vi "Load IBW File.vi"(2 "Page":i32=1, 3 "file path (dialog if empty)":path=path "Q:/inst/AFM Drift/SAA00010002.ibw") -> (0 "Image":T1(plugin-control), 1 "Wave Note":string="ScanSize: 4e-06\rFastScanSize: 4e-06\rSlowScanSize: 4e-06\rScanRate: 1.0016\rXOffset: -4.35e-06\rYOffset: -8.3777e-06\rPointsLines: 128\rScanPoints: 128\rScanLines: 128\rScanAngle: 0\rImagingMode:Contact\rInvOLS: 1e-07\rSpringConstant: 1\rAmpInvOLS: 1.09e-07\rFastRatio: 1\rSlowRatio: 1\rTopLine: 255\rBottomLine: 0\rScanMode:Closed Loop\rNapMode:Off\rFMapScanTime: 17.231\rFMapScanPoints: 32\rFMapScanLines: 32\rFMapXYVelocity: 8e-05\rFMapBookWise: 0\rChannel1DataType: 1\rDataTypeSum: 21\rPhaseOffset: 123.8\rPhaseOffset1: 0\rNapPhaseOffset: 123.8\rVoltageParm: 0\rNapParms: 0\r32 bit channel:Height\rReal Parms: End\rInitial Parms: Start\rScanSize: 4e-06\rFastScanSize: 4e-06\rSlowScanSize: 4e-06\rScanRate: 1.0016\rScanSpeed: 1.0016e-05\rXOffset: -4.35e-06\rYOffset: -8.3777e-06\rScanPoints: 128\rScanLines: 128\rRoundFactor: 0.04\rIntegralGain: 48.62\rProportionalGain: 0\rScanAngle: 0\rScanAngleFactor: 1\rAmplitudeSetpointVolts: 0.54\rAmplitudeSetpointMeters: 1e-08\rDriveAmplitude: 6.4121\rDriveFrequency: 49841\rSweepWidth: 5000\rSlowScanEnabled: 1\rDeflectionSetpointVolts: -0.04\rDeflectionSetpointMeters: 0\rDeflectionSetpointNewtons: 5e-09\rImagingMode: 0\rMaxScanSize: 9e-05\rInvOLS: 1e-07\rSpringConstant: 1\rDisplaySpringConstant: 1e-09\rScanStateChanged: 0\rScanDown: 1\rXLVDTSens: 7.5725e-06\rYLVDTSens: 7.2348e-06\rZLVDTSens: 1.3012e-06\rXLVDTOffset: -0.34\rYLVDTOffset: -0.51\rZLVDTOffset: 0\rYIgain: 8.55\rYPgain: -inf\rXIgain: 8.9531\rXPgain: -inf\rLastScan: 0\rXPiezoSens: 3.8579e-07\rYPiezoSens: 3.9432e-07\rZPiezoSens: 6.8805e-08\rXDriveOffset: 0\rYDriveOffset: 0\rSweepPoints: 480\rSecretGain: 0\rYSgain: 10.5\rXSgain: 10.95\rDIsplayLVDTTraces: 0\rPhaseOffset: 123.8\rBaseSuffix: 2\rSaveImage: 2\rParmChange: 0\rADCgain: 0\rOldADCgain: 12\rOldScanSize: NaN\rOldYOffset: -8.3777e-06\rOldXOffset: -4.3966e-06\rZIgain: 10.15\rZPgain: -inf\rZSgain: 0\rAmpInvOLS: 1.09e-07\rUpdateCounter: 0\rDoMunge: 0\rXMungeAlpha: 1\rYMungeAlpha: 1\rZMungeAlpha: 1\rStartHeadTemp: 33.375 °C\rStartScannerTemp: 26.938 °C\rHas1xACDeflGain: 1\rDontChangeXPT: 0\rLowNoise: 1\rScreenRatio: 0.75\rXDriftRate: 0\rYDriftRate: 0\rXDriftTotal: 0\rYDriftTotal: 0\rDriftBIts: 0\rDriftCount: 0\rSetpoint: 0.0008\rFastRatio: 1\rSlowRatio: 1\rTopLine: 255\rBottomLine: 0\rScanStatus: 1\rIs1DPlus: 0\rDelayUpdate: 0\rMarkerRatio: 0\rStartLineCount: 128\rOldAmplitudeSetpointVolts: 0.54\rOldDeflectionSetPointVolts: 0\rScanMode: 0\rInterpolate: -624\rTipVoltage: 0\rStartHeaterTemp: 0 °C\rEndHeaterTemp: 0\rSurfaceVoltage: 0\rFreqIgain: 5\rFreqPgain: 0\rFreqSgain: 0\rOrcaGain: NaN\rFreqGainOn: 0\rUserIn0Gain: 1\rUserIn1Gain: 1\rUserIn2Gain: 1\rLateralGain: 1\rIsBipolar: 0\rFrequencyHack: 0\rMagneticField: 0\rDriveGainOn: 0\rDriveIGain: 0\rDrivePGain: 0\rDriveSGain: 0\rUserIn0Offset: 0\rUserIn1Offset: 0\rUserIn2Offset: 0\rLateralOffset: 0\rLastImage: 0\rZoomSize: 0\rZoomXOffset: -4.3966e-06\rZoomYOffset: -8.3777e-06\rUser0Voltage: 0\rUser1Voltage: 0\rExtendedZ: 0\rDriveAmplitude1: 0.1\rDriveFrequency1: 0\rSweepWidth1: 5000\rPhaseOffset1: 0\rAmp2InvOLS: 2e-08\rVoltageParm: 0\rMicroscopeID: 3\rCapacitanceSens: 1\rCapacitanceOffset: 0\rCapPhaseOffset: 0\rTipBiasOffset: 0\rTipHeaterOffset: 0\rSurfaceBiasOffset: 0\rUseCantHolder: 0\rCurrentCantHolder: 2\rHasClickRing: 0\rXScanDirection: 1\rYScanDirection: 1\rSaveImageCount: 0\rSaveImageLines: 64\rOrcaGain2: NaN\rUpdateSlowWave: 0\rFBFilterBW: 1000\rCurrentSetpointAmps: 1\rCurrentSetpointVolts: 1\rOldCurrentSetpointVolts: 1\rOldCurrentSetpointAmps: 1\rHasFM: 1\rLastScanWithdraw: 1\rHasLaserRelay: 0\rToggleLaserRelay: 0\rDecimation: 156\rDARTIGain: 5.5\rDARTPGain: 0\rSampleHolder: 1\rManualSampleHolder: 0\rCypherXPTLock: 0\rXPTLock: 2048\rLogFeedback: 0\rARSysScanBusy: 0\rSimpleControls: 0\rPointsLines: 128\rFreeAirAmplitude: NaN\rFreeAirPhase: NaN\rFreeAirDeflection: -0.14617\rFreeAirDriveAmplitude: 0\rContinualRetune: 0\rForceFilter: 0\rTemperatureSens: 1\rTemperatureOffset: 0\rOffsetBehavior: 0\rInputRange: 10\rXLVDTSensSlope: 0\rYLVDTSensSlope: 0\rXLVDTSensIntercept: 0\rYLVDTSensIntercept: 0\rHaveWeKilledTheProgressBar: 0\rPreScanSetting: 0\rImageFrameTime: 0\rMicroscopeModel:MFP3D\rInitial Parms: End\rNapIntegralGain: 10\rNapProportionalGain: 0\rNapDeflectionSetpointVolts: 0.5\rNapAmplitudeSetpointVolts: 0.8\rNapDissipationSetpointVolts: 0.2\rNapFrequencySetPointHz: 0\rNapCurrentSetpointAmps: 1\rNapDriveAmplitude: 1\rNapDriveFrequency: 49797\rNapDriveAmplitude1: 0.1\rNapDriveFrequency1: 4.2e+05\rNapPhaseOffset: 90\rNapTipVoltage: 3\rNapSurfaceVoltage: 0\rNapUser0Voltage: 0\rNapUser1Voltage: 0\rNapHeight: 5e-08\rNapStartHeight: 0\rNapTime: 0.10016\rNapMode: 0\rNapParms: 0\rPotentialIGain: 3\rPotentialPGain: 0\rPotentialGainOn: 0\rElectricTune: 0\rNapCurrentSetpointVolts: 1\rPotentialLoopLimit: 9\rChannel1DataType: 1\rChannel2DataType: 3\rChannel3DataType: 5\rChannel4DataType: 0\rChannel5DataType: 0\rChannel6DataType: 0\rDataTypeSum: 21\rChannel1Show: 2\rChannel2Show: 2\rChannel3Show: 2\rChannel4Show: 2\rChannel5Show: 2\rChannel6Show: 1\rChannelShowSum: 7\rRealPlanefit: 2\rSavePlanefit: 0\rHeightCapture: 2\rHeight1DataScale: 1.2e-09\rHeight1DataOffset: 0\rHeight1RealPlanefit: 2\rHeight1SavePlanefit: 4\rHeight1ColorMap: 2\rHeight2DataScale: 5e-08\rHeight2DataOffset: 0\rHeight2RealPlanefit: 2\rHeight2SavePlanefit: 2\rHeight2ColorMap: 1\rDeflectionCapture: 2\rDeflection1DataScale: 1e-08\rDeflection1DataOffset: 0\rDeflection1RealPlanefit: 1\rDeflection1SavePlanefit: 0\rDeflection1ColorMap: 1\rDeflection2DataScale: 1e-08\rDeflection2DataOffset: 0\rDeflection2RealPlanefit: 2\rDeflection2SavePlanefit: 2\rDeflection2ColorMap: 1\rAmplitudeCapture: 2\rAmplitude1DataScale: 1.5e-10\rAmplitude1DataOffset: -0\rAmplitude1RealPlanefit: 1\rAmplitude1SavePlanefit: 0\rAmplitude1ColorMap: 9\rAmplitude2DataScale: 2e-08\rAmplitude2DataOffset: 0\rAmplitude2RealPlanefit: 1\rAmplitude2SavePlanefit: 2\rAmplitude2ColorMap: 1\rZSensorCapture: 2\rZSensor1DataScale: 8.4e-08\rZSensor1DataOffset: -0\rZSensor1RealPlanefit: 4\rZSensor1SavePlanefit: 2\rZSensor1ColorMap: 1\rZSensor2DataScale: 60\rZSensor2DataOffset: 0\rZSensor2RealPlanefit: 2\rZSensor2SavePlanefit: 2\rZSensor2ColorMap: 1\rPhaseCapture: 2\rPhase1DataScale: 7.5\rPhase1DataOffset: 69.5\rPhase1RealPlanefit: 0\rPhase1SavePlanefit: 0\rPhase1ColorMap: 9\rPhase2DataScale: 60\rPhase2DataOffset: 0\rPhase2RealPlanefit: 2\rPhase2SavePlanefit: 2\rPhase2ColorMap: 1\rOffCapture: 2\rOff1DataScale: 1\rOff1DataOffset: 0\rOff1RealPlanefit: 2\rOff1SavePlanefit: 2\rOff1ColorMap: 9\rOff2DataScale: 0\rOff2DataOffset: 0\rOff2ColorMap: 1\rUserIn1Capture: 2\rUserIn11DataScale: 1\rUserIn11DataOffset: 0\rUserIn11RealPlanefit: 0\rUserIn11SavePlanefit: 0\rUserIn11ColorMap: 1\rUserIn12DataScale: 1\rUserIn12DataOffset: 0\rUserIn12RealPlanefit: 2\rUserIn12SavePlanefit: 2\rUserIn12ColorMap: 1\rUserIn2Capture: 2\rUserIn21DataScale: 1\rUserIn21DataOffset: 0\rUserIn21RealPlanefit: 0\rUserIn21SavePlanefit: 0\rUserIn21ColorMap: 1\rUserIn22DataScale: 1\rUserIn22DataOffset: 0\rUserIn22RealPlanefit: 2\rUserIn22SavePlanefit: 2\rUserIn22ColorMap: 1\rUserIn0Capture: 2\rUserIn01DataScale: 1\rUserIn01DataOffset: 0\rUserIn01RealPlanefit: 0\rUserIn01SavePlanefit: 0\rUserIn01ColorMap: 1\rUserIn02DataScale: 1\rUserIn02DataOffset: 0\rUserIn02RealPlanefit: 2\rUserIn02SavePlanefit: 2\rUserIn02ColorMap: 1\rInputICapture: 2\rInputI1DataScale: 1\rInputI1DataOffset: 0\rInputI1RealPlanefit: 0\rInputI1SavePlanefit: 0\rInputI1ColorMap: 1\rInputI2DataScale: 1\rInputI2DataOffset: 0\rInputI2RealPlanefit: 2\rInputI2SavePlanefit: 2\rInputI2ColorMap: 1\rInputQCapture: 2\rInputQ1DataScale: 1\rInputQ1DataOffset: 0\rInputQ1RealPlanefit: 0\rInputQ1SavePlanefit: 0\rInputQ1ColorMap: 1\rInputQ2DataScale: 1\rInputQ2DataOffset: 0\rInputQ2RealPlanefit: 2\rInputQ2SavePlanefit: 2\rInputQ2ColorMap: 1\rLateralCapture: 2\rLateral1DataScale: 0.01\rLateral1DataOffset: 0\rLateral1RealPlanefit: 1\rLateral1SavePlanefit: 0\rLateral1ColorMap: 1\rLateral2DataScale: 1\rLateral2DataOffset: 0\rLateral2RealPlanefit: 2\rLateral2SavePlanefit: 2\rLateral2ColorMap: 1\rFrequencyCapture: 0\rFrequency1DataScale: 1\rFrequency1DataOffset: 0\rFrequency1RealPlanefit: 1\rFrequency1SavePlanefit: 0\rFrequency1ColorMap: 1\rFrequency2DataScale: 1\rFrequency2DataOffset: 0\rFrequency2RealPlanefit: 2\rFrequency2SavePlanefit: 2\rFrequency2ColorMap: 1\rCurrentCapture: 2\rCurrent1DataScale: 1e-09\rCurrent1DataOffset: 0\rCurrent1RealPlanefit: 0\rCurrent1SavePlanefit: 0\rCurrent1ColorMap: 1\rCurrent2DataScale: 1e-09\rCurrent2DataOffset: 0\rCurrent2RealPlanefit: 2\rCurrent2SavePlanefit: 2\rCurrentColorMap: 1\rCurrent2Capture: 2\rCurrent21DataScale: 1e-06\rCurrent21DataOffset: 0\rCurrent21RealPlanefit: 0\rCurrent21SavePlanefit: 0\rCurrent21ColorMap: 1\rCurrent22DataScale: 1e-06\rCurrent22DataOffset: 0\rCurrent22RealPlanefit: 0\rCurrent22SavePlanefit: 0\rCurrent22ColorMap: 1\rUserCalcCapture: 2\rUserCalc1DataScale: 1\rUserCalc1DataOffset: 0\rUserCalc1RealPlanefit: 2\rUserCalc1SavePlanefit: 2\rUserCalc1ColorMap: 1\rUserCalc2DataScale: 1\rUserCalc2DataOffset: 0\rUserCalc2RealPlanefit: 2\rUserCalc2SavePlanefit: 2\rUserCalc2ColorMap: 1\rCountCapture: 2\rCount1DataScale: 1\rCount1DataOffset: 0\rCount1RealPlanefit: 0\rCount1SavePlanefit: 0\rCount1ColorMap: 1\rCount2DataScale: 1\rCount2DataOffset: 0\rCount2RealPlanefit: 2\rCount2SavePlanefit: 2\rCount2ColorMap: 1\rPotentialCapture: 0\rPotential1DataScale: 1\rPotential1DataOffset: 0\rPotential1RealPlanefit: 0\rPotential1SavePlanefit: 0\rPotential1ColorMap: 1\rPotential2DataScale: 1\rPotential2DataOffset: 0\rPotential2RealPlanefit: 2\rPotential2SavePlanefit: 2\rPotential2ColorMap: 1\rAmplitude1Capture: 2\rAmplitude11DataScale: 2e-08\rAmplitude11DataOffset: 0\rAmplitude11RealPlanefit: 1\rAmplitude11SavePlanefit: 0\rAmplitude11ColorMap: 9\rAmplitude12DataScale: 2e-08\rAmplitude12DataOffset: 0\rAmplitude12RealPlanefit: 1\rAmplitude12SavePlanefit: 2\rAmplitude12ColorMap: 1\rAmplitude2Capture: 2\rAmplitude21DataScale: 2e-08\rAmplitude21DataOffset: 0\rAmplitude21RealPlanefit: 1\rAmplitude21SavePlanefit: 0\rAmplitude21ColorMap: 9\rAmplitude22DataScale: 2e-08\rAmplitude22DataOffset: 0\rAmplitude22RealPlanefit: 1\rAmplitude22SavePlanefit: 2\rAmplitude22ColorMap: 1\rPhase1Capture: 2\rPhase11DataScale: 60\rPhase11DataOffset: 90\rPhase11RealPlanefit: 0\rPhase11SavePlanefit: 0\rPhase11ColorMap: 9\rPhase12DataScale: 60\rPhase12DataOffset: 0\rPhase12RealPlanefit: 2\rPhase12SavePlanefit: 2\rPhase12ColorMap: 1\rPhase2Capture: 2\rPhase21DataScale: 60\rPhase21DataOffset: 90\rPhase21RealPlanefit: 0\rPhase21SavePlanefit: 0\rPhase21ColorMap: 9\rPhase22DataScale: 60\rPhase22DataOffset: 0\rPhase22RealPlanefit: 2\rPhase22SavePlanefit: 2\rPhase22ColorMap: 1\rChannel1Scope: 3\rChannel2Scope: 3\rChannel3Scope: 3\rChannel4Scope: 3\rChannel5Scope: 3\rChannel6Scope: 0\rChannel1Auto: 1\rChannel2Auto: 1\rChannel3Auto: 1\rChannel4Auto: 1\rChannel5Auto: 1\rChannel6Auto: 0\rChannel1AutoImg: 0\rChannel2AutoImg: 0\rChannel3AutoImg: 0\rChannel4AutoImg: 0\rChannel5AutoImg: 0\rUserCalcFunc: 1\rDissipationCapture: 2\rDissipation1DataScale: 0.1\rDissipation1DataOffset: 0\rDissipation1RealPlanefit: 1\rDissipation1SavePlanefit: 0\rDissipation1ColorMap: 1\rDissipation2DataScale: 1\rDissipation2DataOffset: 0\rDissipation2RealPlanefit: 2\rDissipation2SavePlanefit: 2\rDissipation2ColorMap: 1\rFixOffset: 0\rInA: Ground\rInB: Ground\rInFast: FilterOut\rInAOffset: Ground\rInBOffset: Ground\rInFastOffset: Ground\rOutXMod: Off\rOutYMod: Off\rOutZMod: Off\rFilterIn: Defl\rBNCOut0: Ground\rBNCOut1: ACDefl\rBNCOut2: Ground\rPogoOut: Ground\rChip: Ground\rShake: DDS\rInput.Z.Filter.Freq: 2000\rInput.X.Filter.Freq: 1000\rInput.Y.Filter.Freq: 1000\rInput.A.Filter.Freq: 2000\rInput.B.Filter.Freq: 2000\rInput.Fast.Filter.Freq: 1500\rLockin.0.Filter.Freq: 1000\rLockin.1.Filter.Freq: 1000\rThermalDC: 1e-14\rThermalQ: 20\rThermalFrequency: 49797\rThermalWhiteNoise: 5e-15\rScaleLog: 3\rFitWidth: 20000\rThermalSamples: 1000\rThermalCounter: 0\rSectionSamples: 10\rSectionCounter: 0\rDoThermal: 0\rThermalResolution: 4\rThermalZoom: 0\rDoCantTune: 0\rZoomCounter: 200\rAutoTuneLow: 10000\rAutoTuneHigh: 1e+05\rTargetVoltage: 0.8\rTargetPercent: -5\rCheckTuneTraces: 0\rButtonTime: 1.0155e+09\rShowThermalFit: 0\rAppendThermalBit: 8\rTuneQ: 100\rTuneGain: 0\rTunePeakResult: 0.8271\rTuneFreqResult: 49914\rTuneQResult: 102.68\rThermalSamplesLimit: 0\rTuneFeedback: 0\rTuneDDSOutput: 0\rTipVoltCenter: 0\rTipVoltWidth: 10\rThermalFrequencyRange: 2\rAutoTuneLimit: 0\rAutoTuneLow1: 3e+05\rAutoTuneHigh1: 6e+05\rTargetVoltage1: 0.1\rTargetPercent1: 0\rDualACMode: 0\rWhichACMode: 0\rBackwardsTune: 0\rTuneCaptureRate: 500\rTuneTime: 0.96\rTuneFilter: 500\riDriveOn: 0\rFrequencyRatio: 0\rDFRTFrequencyCenter: 3.5e+05\rDFRTFrequencyWidth: 5000\rDFRTOn: 0\rThermalCenter: 49797\rThermalWidth: 30000\rDFWMAMT: 0\rLastXPos: 0\rLastYPos: 0\rPFMFrequencyLimit: inf\rTuneLockin: 0\rTipHeaterDrive: 0\rAdjustSpringConstant: 1\rDrawThermalFit: 0\rLateralTune: 0\rThermalTemperature: 298\rUseCypherThermal: 0\rUseCypherMultiThread: 0\rIllumination: 0\rTuneAngle: 0\rIsDefaultFrequency: 0\rLossTanAmp1: 0.8032\rLossTanPhase1: 67.462\rLossTanAmp2: 0.0089164\rLossTanPhase2: -48.104\rLossTanFreq1: 49841\rLossTanFreq2: 0\rLossTanQ1: 102.68\rLossTanQ2: 0\rYourVariablesStartHere: 0\rLog File:Start\rLog File:Stop\rDate:2013-11-10\rTime:12:57:43 PM\rSeconds:3466933064\rUserCalcUnit: °\rUserIn0Unit: V\rUserIn1Unit: V\rUserIn2Unit: V\rLateralUnit: V\rARUserPanelName: \rUserIn0Name: \rUserIn1Name: \rUserIn2Name: \rUserCalcName: \rUserIn0Ab: \rUserIn1Ab: \rUserIn2Ab: \rUserCalcAb: \rUserIn0Force: \rUserIn1Force: \rUserIn2Force: \rUserCalcForce: \rSaveImage: E:Users:Shicheng:20131110:\rSaveForce: E:Users:Shicheng:20131110:\rLastSaveImage: E:Users:Shicheng:20131110:\rLastSaveForce: E:Users:Shicheng:20131110:\rNavLoadPath: \rLastNavLoadPath: \rDetectorSum: Head.Laser.Sum\rXSensor: Input.X\rYSensor: Input.Y\rZSensor: Input.Z\rDDSAmplitude0: $Lockin.0.Amp\rDDSDCOffset0: $Lockin.DCOffset\rDDSFrequency0: $Lockin.0.Freq\rDDSFrequencyOffset0: $Lockin.0.FreqOffset\rDDSPhaseOffset0: $Lockin.0.PhaseOffset\rDDSAmplitude1: $Lockin.1.Amp\rDDSFrequency1: $Lockin.1.Freq\rDDSPhaseOffset1: $Lockin.1.PhaseOffset\rAmplitude: $Lockin.0.r\rPhase: $Lockin.0.theta\rInputi: $Lockin.0.i\rInputq: $Lockin.0.q\rDissipation: $DDSAmplitude0\rCount: Input.Counter\rPotential: $DDSDCOffset0\rAmplitude1: $Lockin.1.r\rPhase1: $Lockin.1.theta\rDeflection: Input.Fast\rLateral: Head.Laser.Lateral\rFrequency: $DDSFrequencyOffset0\rLockIn: ARC.Lockin\rHeight: output.Z\rHeightLoop: PIDSloop.2\routputXLoop: PIDSloop.0\routputYLoop: PIDSloop.1\rVerDate:101010.1202\rVersion:101010+1202\rXopVersion:20102.29.21.0\rOSVersion:Windows 7 Professional Service Pack 1 (Build 7601)\rIgorFileVersion:6.3.1.2\rBaseName:SAA0001\rImageNote:\rTipSerialNumber:\r\rPlanefit 0: Flatten 1\rPlanefitOrder 0: -1\rFlattenOrder 0: 1\rPlanefit Offset 0: -3.6389e-07\rPlanefit X Slope 0: 0\rPlanefit Y Slope 0: 0\rFlatten Offsets 0: -3.09680871e-07,-3.094801e-07,-3.09203273e-07,-3.08500148e-07,-3.08303385e-07,-3.07591392e-07,-3.07790998e-07,-3.07644797e-07,-3.07800121e-07,-3.07523322e-07,-3.08123532e-07,-3.08585953e-07,-3.08692506e-07,-3.09404612e-07,-3.09369511e-07,-3.0876717e-07,-3.09760253e-07,-3.10183282e-07,-3.10542276e-07,-3.10926936e-07,-3.11413402e-07,-3.11160591e-07,-3.11844332e-07,-3.11971291e-07,-3.12337704e-07,-3.12449799e-07,-3.11962992e-07,-3.12703179e-07,-3.12881241e-07,-3.12356804e-07,-3.12051583e-07,-3.1401558e-07,-3.13279344e-07,-3.1341645e-07,-3.12781395e-07,-3.09348565e-07,-3.08705097e-07,-3.02255359e-07,-3.05831179e-07,-3.09353794e-07,-3.19753639e-07,-3.26000389e-07,-3.25950651e-07,-3.25856519e-07,-3.25715149e-07,-3.25609392e-07,-3.2544375e-07,-3.25418483e-07,-3.25386225e-07,-3.25494142e-07,-3.26036115e-07,-3.25817524e-07,-3.25752126e-07,-3.25552804e-07,-3.25845065e-07,-3.25858053e-07,-3.26744754e-07,-3.2748585e-07,-3.27761427e-07,-3.28567523e-07,-3.28968326e-07,-3.29388996e-07,-3.29970305e-07,-3.29905816e-07,-3.29505184e-07,-3.29136583e-07,-3.28694568e-07,-3.28580086e-07,-3.27844191e-07,-3.27600617e-07,-3.2738393e-07,-3.27476016e-07,-3.26845537e-07,-3.26557995e-07,-3.26427767e-07,-3.2659247e-07,-3.26949959e-07,-3.23217137e-07,-3.24136323e-07,-3.24881881e-07,-3.25219673e-07,-3.25950055e-07,-3.26396759e-07,-3.27009673e-07,-3.2757481e-07,-3.28054995e-07,-3.28594439e-07,-3.28868396e-07,-3.29464882e-07,-3.29918066e-07,-3.30559118e-07,-3.31161402e-07,-3.31429931e-07,-3.32143657e-07,-3.32802983e-07,-3.33638468e-07,-3.34399658e-07,-3.34783095e-07,-3.34843804e-07,-3.35126714e-07,-3.34999498e-07,-3.35852263e-07,-3.35845669e-07,-3.36798422e-07,-3.368215e-07,-3.37227362e-07,-3.37833512e-07,-3.38673061e-07,-3.39432688e-07,-3.40166878e-07,-3.40839591e-07,-3.41987004e-07,-3.43397886e-07,-3.44311388e-07,-3.45346535e-07,-3.46683237e-07,-3.48134336e-07,-3.4980755e-07,-3.51813412e-07,-3.54007454e-07,-3.56376518e-07,-3.58599891e-07,-3.61383798e-07,-3.6436586e-07,-3.68601548e-07,-3.73615109e-07,-3.78952791e-07,-3.89368125e-07,\rFlatten Slopes 0: -0.0211464316,-0.0211897157,-0.0211820994,-0.0214031171,-0.0215037428,-0.0217332449,-0.0216206871,-0.0216016509,-0.0215143915,-0.0217771456,-0.0217752736,-0.0216612089,-0.0218268428,-0.0216768924,-0.0216035135,-0.022035148,-0.0219925307,-0.021867061,-0.0218446776,-0.0218969565,-0.0217439085,-0.0219007581,-0.0218512025,-0.0218427535,-0.0217134878,-0.021713214,-0.0218732916,-0.0217641294,-0.0216180719,-0.0217579622,-0.0217983127,-0.0200188868,-0.0218776036,-0.0220667347,-0.022236174,-0.0237909667,-0.0241756365,-0.0267515406,-0.0255619287,-0.0243461765,-0.0187465437,-0.0166872181,-0.016711235,-0.0166833531,-0.0166600514,-0.0166439787,-0.0167258754,-0.0166074876,-0.0167064648,-0.0168481655,-0.0166732166,-0.0167105515,-0.0166866351,-0.0167223774,-0.0166781005,-0.0167811569,-0.0167170595,-0.0167105943,-0.0167626794,-0.016734289,-0.016697064,-0.0167137738,-0.0166197587,-0.0166322514,-0.016608024,-0.0165972337,-0.0166405383,-0.0165562518,-0.0166794229,-0.0166673865,-0.0166751072,-0.0165979788,-0.0166732371,-0.0166071989,-0.0166615471,-0.0167553965,-0.0167266931,-0.016809376,-0.0167572442,-0.0167033486,-0.0167792458,-0.0167003963,-0.0168231744,-0.0167986751,-0.0167197809,-0.0167437866,-0.0166525599,-0.0167138372,-0.0167670716,-0.0166877974,-0.016725773,-0.0166745503,-0.0167281851,-0.0167071912,-0.0166910384,-0.0167091358,-0.0166698545,-0.0165723208,-0.0166240968,-0.0165717769,-0.0166536756,-0.0164471958,-0.0166992899,-0.0165543724,-0.0166396536,-0.0166763589,-0.0167526025,-0.0167055205,-0.0166565161,-0.0166519377,-0.0166681446,-0.0167054012,-0.0166759007,-0.0167079885,-0.0167815238,-0.0167457331,-0.0166667718,-0.0167129654,-0.0167109035,-0.0167416073,-0.0167334285,-0.0167379454,-0.0167797338,-0.0168992803,-0.016864771,-0.0169978905,-0.0171406735,-0.0178104974,\rDisplay Offset 0: 0\rDisplay Range 0: 1.2e-09\rColorMap 0: Grays256\rPlanefit 1: None\rPlanefitOrder 1: -1\rFlattenOrder 1: -1\rPlanefit Offset 1: 0\rPlanefit X Slope 1: 0\rPlanefit Y Slope 1: 0\rDisplay Offset 1: -3.9615e-09\rDisplay Range 1: 1e-08\rColorMap 1: Grays256\rPlanefit 2: Planefit\rPlanefitOrder 2: 1\rFlattenOrder 2: -1\rPlanefit Offset 2: -1.5419e-06\rPlanefit X Slope 2: -0.017946\rPlanefit Y Slope 2: 0.0069998\rDisplay Offset 2: 0\rDisplay Range 2: 8.4e-08\rColorMap 2: Grays256\rEndHeadTemp:33.375 °C\rEndScannerTemp:26.9375 °C\r")   [LabVIEW 2013]
uses:
  <vilib>/vision/NI_Vision_Development_Module.lvlib
panel:
  out "error out":errorcluster
  in  "Type of Symmetry":u32(ring) items=["Horizontal", "Vertical", "Central", "1st Diagonal", "2nd Diagonal"]
  out "Wave Name":string
  in  "Array":i8[](array[numeric])
  out "Wave Created":timestamp=timestamp(3373459566 s since 1904-01-01) format="%<%.3X\n%Y/%m/%d>T"
  in  "dates and points":T2
  in  "Array 2":i8[](array[numeric])
  out "Output Array":dbl[][][](array[numeric])
  out "Intensity Graph":sgl[][](graph)
  in  "Cluster":T3
  out "dim size":i32[](array[numeric])=[128, 128, 3, 0]
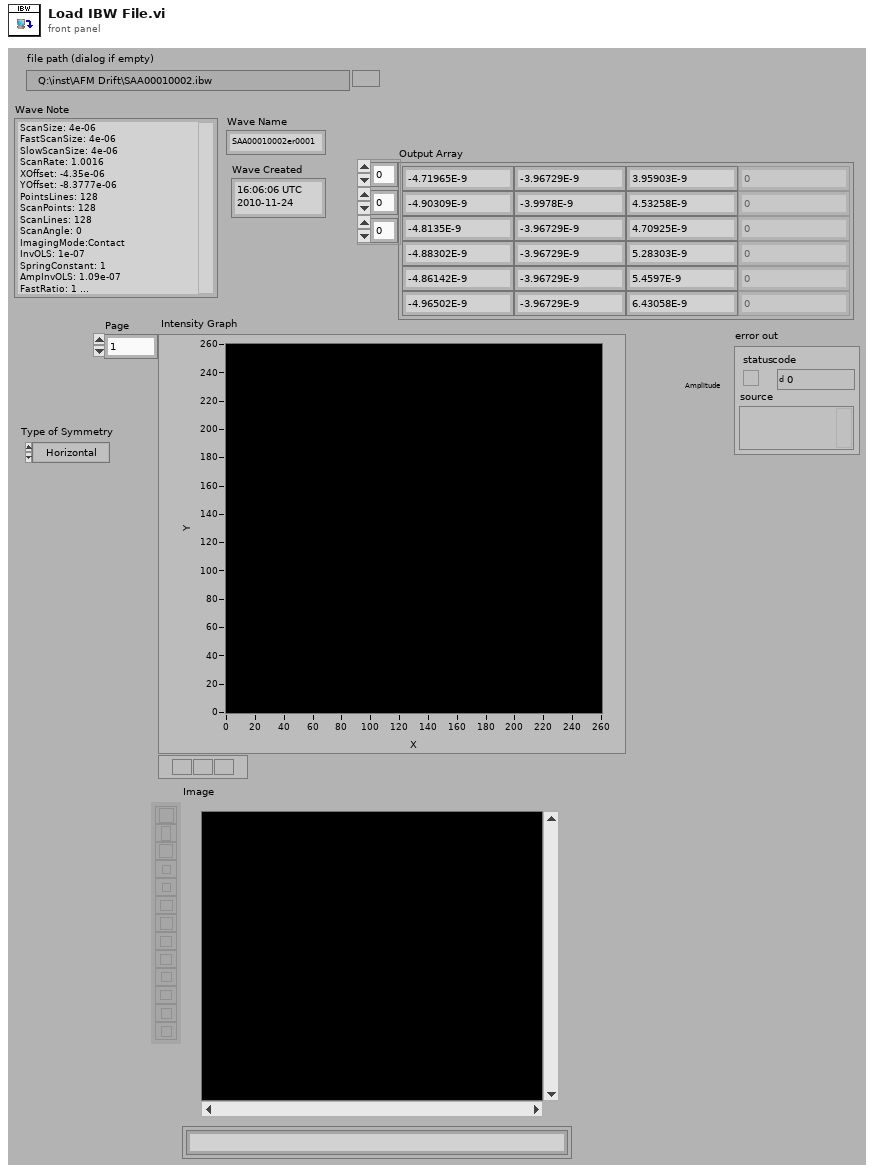
[diagram p1: front panel]
types:
  T1 = typedef "IMAQ Image.ctl" = refnum<image>
  T2 = cluster{"creation date":u32, "mod date":u32, "nmpnts":i32, "type":i16}
  T3 = cluster{"version":i16, "checksum":i16, "wfmSize":i32, "formulaSize":i32, "noteSize":i32}
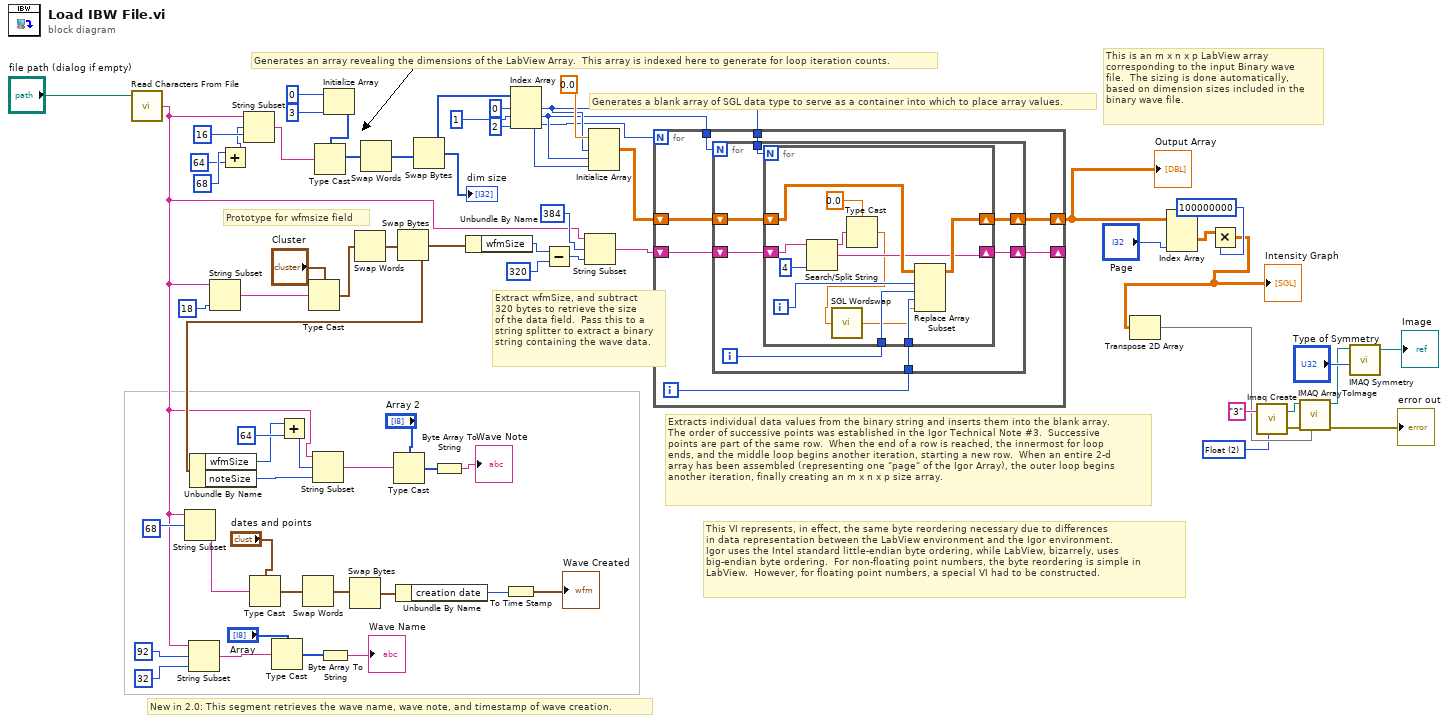
[diagram p0: block diagram]
diagram:
  w1 = u32 2 items=["8 bits", "16 bits", "Float", "Complex", "RGB", "HSL"] ("Image Type")
  # "New in 2.0: This segment retrieves the wave name, wave note, and timestamp of wave creation."
  # "This VI represents, in effect, the same byte reordering necessary due to differences\nin data representation between the LabView environment and the Igor environment.\nIgor uses the Intel standard little-endian byte ordering, while LabView, bizarrely, uses\nbig-endian byte ordering.  For non-floating point numbers, the byte reordering is simple in\nLabView.  However, for floating point numbers, a special VI had to be constructed."
  # "This is an m x n x p LabView array\ncorresponding to the input Binary wave\nfile.  The sizing is done automatically,\nbased on dimension sizes included in the\nbinary wave file."
  # "Generates a blank array of SGL data type to serve as a container into which to place array values."
  # "Extracts individual data values from the binary string and inserts them into the blank array.\nThe order of successive points was established in the Igor Technical Note #3.  Successive\npoints are part of the same row.  When the end of a row is reached, the innermost for loop\nends, and the middle loop begins another iteration, starting a new row.  When an entire 2-d\narray has been assembled (representing one \"page\" of the Igor Array), the outer loop begins\nanother iteration, finally creating an m x n x p size array."
  # "Extract wfmSize, and subtract\n320 bytes to retrieve the size\nof the data field.  Pass this to a\nstring splitter to extract a binary\nstring containing the wave data."
  # "Prototype for wfmsize field"
  # "Generates an array revealing the dimensions of the LabView Array.  This array is indexed here to generate for loop iteration counts."
  n1 = call <vilib>:"Read Characters From File.vi"("file path (dialog if empty)"="file path (dialog if empty)") -> ("character string"=w13:string)  [unwired: 1 in, 7 out]
  n2 = String Subset(string=w13, offset (0)=68 ("nmpnts offset")) -> (substring=w26:string)  [unwired: 1 out]
  n3 = String Subset(string=w13, offset (0)=92 ("wave name offset"), length (rest)=32 ("length (rest)")) -> (substring=w17:string)
  n4 = String Subset(string=w13, length (rest)=18 ("length (rest)")) -> (substring=w60:string)  [unwired: 1 out]
  n5 = Add(x=68 ("dims offset"), y=64) -> (x+y=w46:i32)
  n6 = String Subset(string=w13, offset (0)=w46, length (rest)=16 ("length (rest)")) -> (substring=w65:string)
  n7 = Type Cast(type="dates and points", x=w26) -> (*(type *) &x=w21:T2)
  n8 = Type Cast(type="Array", x=w17) -> (*(type *) &x=w15:i8[])
  n9 = Swap Words(1:w21) -> (0:w20:T2)
  n10 = Type Cast(type="Cluster", x=w60) -> (*(type *) &x=w32:T3)
  n11 = Byte Array To String(unsigned byte array=w15) -> (string=→"Wave Name":string)
  n12 = Initialize Array(0 ("element"), 3 ("dimension size")) -> (w66:i32[])
  n13 = Type Cast(type=w66, x=w65) -> (*(type *) &x=w67:i32[])
  n14 = Swap Bytes(anything=w20) -> (byte swapped=w24:T2)
  n15 = Swap Words(1:w32) -> (0:w62:T3)
  n16 = Swap Words(1:w67) -> (0:w68:i32[])
  n17 = Unbundle By Name(w24) -> ("creation date"=w22:u32)
  n18 = Swap Bytes(anything=w62) -> (byte swapped=w30:T3)
  n19 = Unbundle By Name(w30) -> ("wfmSize"=w29:i32, "noteSize"=w28:i32)
  n20 = Add(x=w29, y=64) -> (x+y=w36:i32)
  n21 = String Subset(string=w13, offset (0)=w36, length (rest)=w28) -> (substring=w35:string)
  n22 = Type Cast(type="Array 2", x=w35) -> (*(type *) &x=w33:i8[])
  n23 = Swap Bytes(anything=w68) -> (byte swapped=w54:i32[])
  "dim size" <- w54
  n24 = Byte Array To String(unsigned byte array=w33) -> (string=→"Wave Note":string)
  n25 = Unbundle By Name(w30) -> ("wfmSize"=w58:i32)
  n26 = To Time Stamp(1:w22) -> (0:→"Wave Created":timestamp)
  n27 = Index Array(array=w54, index #1=0 ("index"), index #2=1 ("index"), index #3=2 ("index")) -> (element #1=w41:i32, element #2=w40:i32, element #3=w39:i32)
  n28 = Subtract(x=w58, y=320) -> (x-y=w56:i32)
  n29 = String Subset(string=w13, offset (0)=384, length (rest)=w56) -> (substring=w43:string)
  n30 = Initialize Array(sgl 0.0 ("element"), w41, w40, w39) -> (w50:sgl[][][])
  n31 = for {
    N: w39 -> [_]
    shift-right: [w71] -> w49
    shift-left: w50 -> [w75]
    shift-right: [w70] -> _
    shift-left: w43 -> [w74]
    tunnel: w41 -> [w73]
    tunnel: w40 -> [w69]
    i -> [w72]
    n32 = for {
      N: w69 -> [_]
      shift-right: [w77] -> w71
      shift-left: w75 -> [w82]
      shift-right: [w76] -> w70
      shift-left: w74 -> [w81]
      tunnel: w73 -> [w80]
      tunnel: w72 -> [w78]
      i -> [w79]
      n33 = for {
        N: w80 -> [_]
        shift-right: [w88] -> w77
        shift-left: w82 -> [w92]
        shift-right: [w87] -> w76
        shift-left: w81 -> [w93]
        tunnel: w79 -> [w90]
        tunnel: w78 -> [w89]
        i -> [w91]
        n34 = Search/Split String(string=w93, offset (0)=4 ("length (rest)")) -> (substring before match=w86:string, match + rest of string=w87:string)  [unwired: 2 out]
        n35 = Type Cast(type=sgl 0.0, x=w86) -> (*(type *) &x=w84:sgl)
        n36 = call "SGL Wordswap.vi"("x"=w84) -> ("*(type *) &x"=w83:sgl)
        n37 = Replace Array Subset(array=w92, new element=w83, index (dim 0)=w91, index (dim 1)=w90, index (dim 2)=w89) -> (w88:sgl[][][])
      }
    }
  }
  "Output Array" <- w49
  n38 = Index Array(array=w49, index (dim 2)="Page") -> (element=w4:sgl[][])  [unwired: 2 in]
  n39 = Multiply(x=w4, y=100000000 ("offset (0)")) -> (x*y=w2:sgl[][])
  "Intensity Graph" <- w2
  n40 = Transpose 2D Array(2D array=w2) -> (transposed array=w5:sgl[][])
  n41 = call "Imaq Create"("Image Name"="3", "Image Type"=w1) -> ("New Image"=w10:T1, "error out"=w9:errorcluster)  [unwired: 2 in, 1 out]
  n42 = call "IMAQ ArrayToImage"("Image Pixels (Float)"=w5, "error in (no error)"=w9, "Image"=w10) -> ("error out"=→"error out":errorcluster, "Image Out"=w7:T1)  [unwired: 3 in, 4 out]
  n43 = call "IMAQ Symmetry"("Type of Symmetry"="Type of Symmetry", "Image Src"=w7) -> ("Image Dst Out"=→"Image":T1)  [unwired: 2 in, 2 out]
